vi "ficheros.vi"() -> ()   [LabVIEW 2020]
uses:
  <vilib>/ErrorRing/Error Ring.xnode
panel:
  in  "Formato":string
  in  "Nombre del Archivo":string
  in  "Ruta de Almacenamiento":path
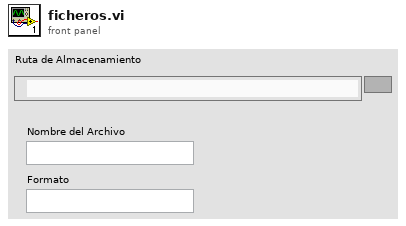
[diagram p1: front panel]
types:
  T1 = enum16{"open", "replace", "create", "open or create", "replace or create", "replace or create with confirmation"}
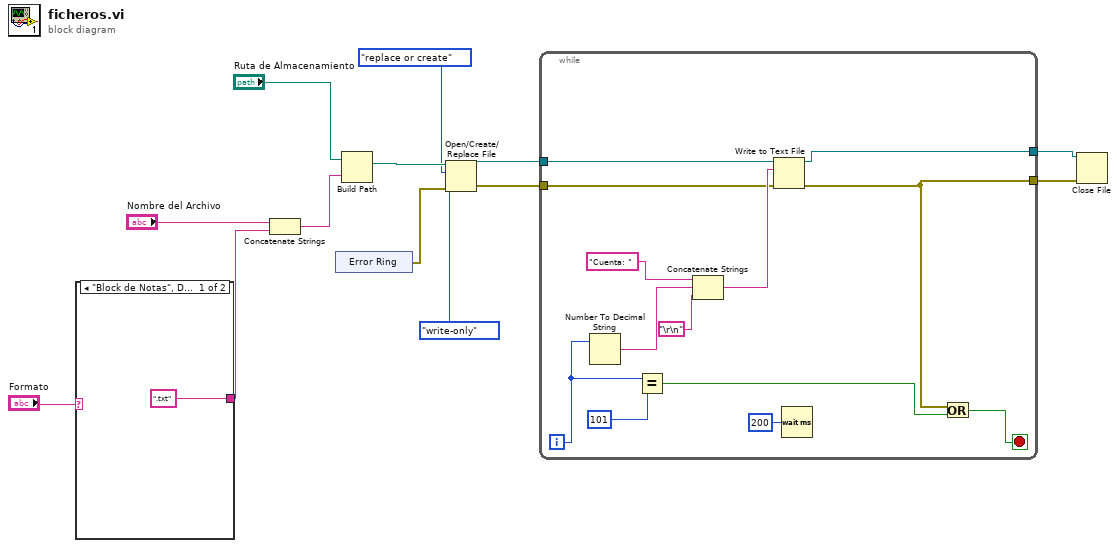
[diagram p0: block diagram]
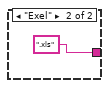
[diagram p2: hidden frame]
diagram:
  n1 = case shown="\"Block de Notas\", Default" "Formato" {
    tunnel: [".txt" ".xls"] -> w9
    frame "Block de Notas", Default {
    }
    frame "Exel" {
    }
  }
  n2 = Concatenate Strings("Nombre del Archivo", w9) -> (w12:string)
  n3 = xnode "Error Ring"() -> ("error out"=w7:errorcluster)
  n4 = Build Path(base path="Ruta de Almacenamiento", name or relative path=w12) -> (appended path=w8:path)
  n5 = Open/Create/Replace File(file path (use dialog)=w8, error in=w7, operation (0:open)=T1."replace or create", access (0:read/write)=enum16{"read/write", "read-only", "write-only"}."write-only") -> (refnum out=w4:refnum<file>, error out=w3:errorcluster)  [unwired: 2 in, 1 out]
  n6 = while {
    tunnel: w4 -> [w19]
    tunnel: w3 -> [w18]
    tunnel: [w17] -> w2
    tunnel: [w16] -> w1
    i -> [w24]
    stop <- w22 stop-if-true
    n7 = Number To Decimal String(number=w24) -> (decimal integer string=w26:string)  [unwired: 1 in]
    n8 = Equal?(x=w24, y=101) -> (x = y?=w21:bool)
    n9 = Concatenate Strings("Cuenta: ", w26, "\r\n") -> (w20:string)
    n10 = Write to Text File(file (use dialog)=w19, text=w20, error in=w18) -> (refnum out=w17:refnum<file>, error out=w16:errorcluster)  [unwired: 1 in, 1 out]
    n11 = Wait (ms)(milliseconds to wait=u32 200) -> ()  [unwired: 1 out]
    n12 = Or(x=w16, y=w21) -> (x .or. y?=w22:bool)
  }
  n13 = Close File(refnum=w2, error in=w1) -> ()  [unwired: 2 out]
